vi "SetDevWorkMode.vi"(8 "错误输入（无错误）":errorcluster, 11 "检波模式索引值":u32) -> (0 "错误输出":errorcluster)   [LabVIEW 2014]
uses:
  X86Dll/ZXUTConfigMgr.dll
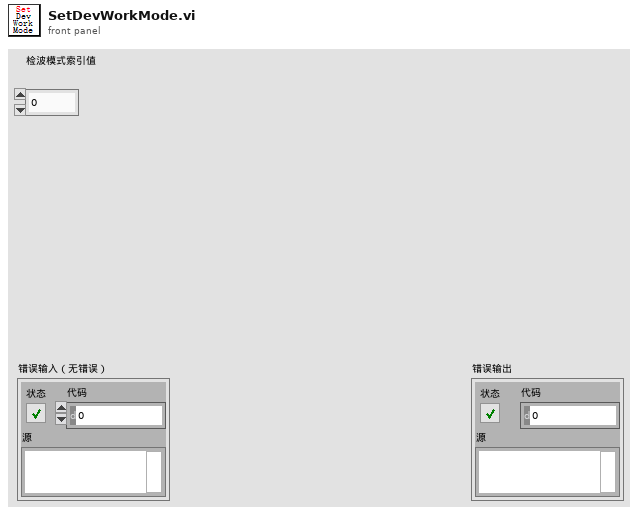
[diagram p1: front panel]
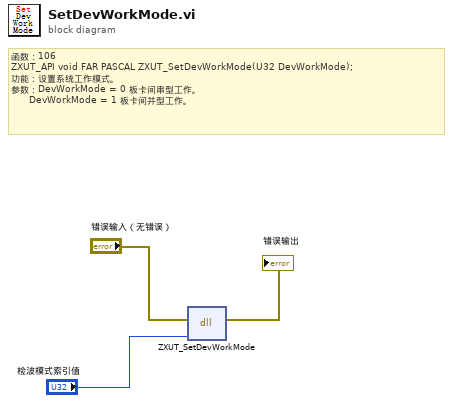
[diagram p0: block diagram]
diagram:
  # "函数：106\nZXUT_API void\tFAR PASCAL ZXUT_SetDevWorkMode(U32 DevWorkMode);\n功能：设置系统工作模式。\n参数：DevWorkMode = 0 板卡间串型工作。\n      DevWorkMode = 1 板卡间并型工作。"
  n1 = dll-call lib="D:/Software/Utrasonic on-line monitoring/X86Dll/ZXUTConfigMgr.dll" fn="ZXUT_SetDevWorkMode"(error in="错误输入（无错误）", "DevWorkMode"="检波模式索引值") -> (error out=→"错误输出":errorcluster)  [unwired: 4 in, 1 out]
